vi "synnax writer open.vi"(4 "enable_auto_commit (F)":bool, 5 "err_on_unauthorized (F)":bool, 6 "auto_index (F)":bool, 7 "start (now)":timestamp, 8 "error in":errorcluster, 9 "authorities (255 for all channels)":u8[](array[numeric]), 10 "channels":u32[](array[numeric]), 11 "sy client handle":u64) -> (0 "error out":errorcluster, 2 "channels out":u32[](array[numeric]), 3 "sy writer handle":u64)   [LabVIEW 2026, in "synnax_clib.lvlib" / "Synnax Writer.lvclass"]
doc: "SYNNAX_EXPORT int32_t synnax_writer_open(\n SynnaxClient client,\n int64_t start,\n const uint32_t *channels,\n uint64_t channel_count,\n int32_t mode,\n int32_t enable_auto_commit,\n SynnaxWriter *out_writer,\n SynnaxError err\n);"
uses:
  Synnax Writer.lvclass
  typedefs/writer_mode.ctl
  subvis/Timestamp Conversion Single.vi
  Synnax Writer.lvclass/Synnax Writer.ctl
  synnax_clib.lvlib
  synnax_clib.dll
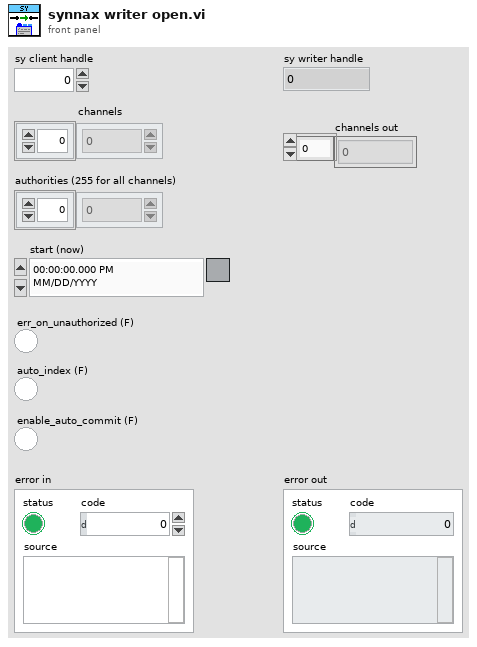
[diagram p1: front panel]
types:
  T1 = typedef "synnax_clib.lvlib/writer_mode.ctl" = enum16{"PERSIST & STREAM", "PERSIST", "STREAM"}
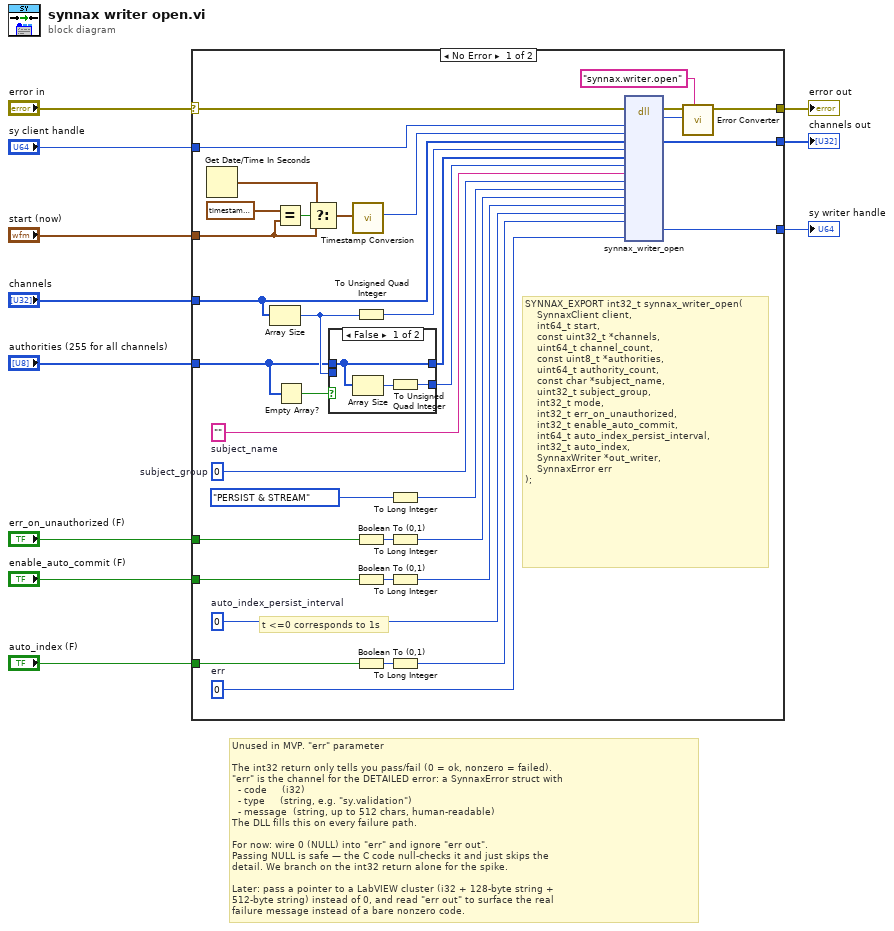
[diagram p0: block diagram]
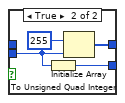
[diagram p2: hidden frame]
diagram:
  # "Unused in MVP. \"err\" parameter\n\nThe int32 return only tells you pass/fail (0 = ok, nonzero = failed).\n\"err\" is the channel for the DETAILED error: a SynnaxError struct with\n  - code     (i32)\n  - type     (string, e.g. \"sy.validation\")\n  - message  (string, up to 512 chars, human-readable)\nThe DLL fills this on every failure path.\n\nFor now: wire 0 (NULL) into \"err\" and ignore \"err out\".\nPassing NULL is safe — the C code null-checks it and just skips the\ndetail. We branch on the int32 return alone for the spike.\n\nLater: pass a pointer to a LabVIEW cluster (i32 + 128-byte string +\n512-byte string) instead of 0, and read \"err out\" to surface the real\nfailure message instead of a bare nonzero code."
  n1 = case shown="No Error" "error in" {
    selector: "error in" -> [w15 w55]
    tunnel: "enable_auto_commit (F)" -> [w47 _]
    tunnel: [w43 w55] -> w10
    tunnel: "err_on_unauthorized (F)" -> [w38 _]
    tunnel: "auto_index (F)" -> [w34 _]
    tunnel: "authorities (255 for all channels)" -> [w27 _]
    tunnel: "start (now)" -> [w13 _]
    tunnel: [w22 _] -> w5
    tunnel: [w21 _] -> w4
    tunnel: "channels" -> [w20 _]
    tunnel: "sy client handle" -> [w19 _]
    frame No Error {
      w35 = i64 0  # auto_index_persist_interval
      w39 = u32 0  # subject_group
      w40 = ""  # subject_name
      w45 = u64 0  # err
      # "t <=0 corresponds to 1s"
      # "SYNNAX_EXPORT int32_t synnax_writer_open(\n    SynnaxClient client,\n    int64_t start,\n    const uint32_t *channels,\n    uint64_t channel_count,\n    const uint8_t *authorities,\n    uint64_t authority_count,\n    const char *subject_name,\n    uint32_t subject_group,\n    int32_t mode,\n    int32_t err_on_unauthorized,\n    int32_t enable_auto_commit,\n    int64_t auto_index_persist_interval,\n    int32_t auto_index,\n    SynnaxWriter *out_writer,\n    SynnaxError err\n);"
      n2 = Get Date/Time In Seconds() -> (seconds since 1Jan1904=w14:timestamp)
      n3 = Array Size(array=w20) -> (size(s)=w30:i32)
      n4 = Equal?(x=timestamp timestamp(0 s since 1904-01-01), y=w13) -> (x = y?=w25:bool)
      n5 = Empty Array?(array=w27) -> (empty?=w28:bool)
      n6 = Select(t=w14, s=w25, f=w13) -> (s? t:f=w24:timestamp)
      n7 = case shown="False" w28 {
        tunnel: [w49 w54] -> w31
        tunnel: w30 -> [_ w52]
        tunnel: w27 -> [w49 _]
        tunnel: [w48 w51] -> w26
        frame False {
          n8 = Array Size(array=w49) -> (size(s)=w50:i32)
          n9 = To Unsigned Quad Integer(1:w50) -> (0:w48:u64)
        }
        frame True {
          n10 = To Unsigned Quad Integer(1:w52) -> (0:w51:u64)
          n11 = Initialize Array(u8 255, w52) -> (w54:u8[])
        }
      }
      n12 = call-poly "Timestamp Conversion.vi"("timestamp"=w24) -> ("timestamp (ns)"=w23:i64)  [unwired: 9 in]
      n13 = To Unsigned Quad Integer(1:w30) -> (0:w29:u64)
      n14 = Boolean To (0,1)(Boolean=w38) -> (0, 1=w37:i16)
      n15 = Boolean To (0,1)(Boolean=w47) -> (0, 1=w46:i16)
      n16 = Boolean To (0,1)(Boolean=w34) -> (0, 1=w33:i16)
      n17 = To Long Integer(number=writer_mode."PERSIST & STREAM") -> (32bit integer=w41:i32)
      n18 = To Long Integer(number=w37) -> (32bit integer=w36:i32)
      n19 = To Long Integer(number=w46) -> (32bit integer=w44:i32)
      n20 = To Long Integer(number=w33) -> (32bit integer=w32:i32)
      n21 = dll-call lib="C/synnax/client/labview/synnax_clib.*" fn="synnax_writer_open"(error in=w15, "client"=w19, "start"=w23, "channels"=w20, "channel_count"=w29, "authorities"=w31, "authority_count"=w26, "subject_name"=w40, "subject_group"=w39, "mode"=w41, "err_on_unauthorized"=w36, "enable_auto_commit"=w44, "auto_index_persist_interval"=w35, "auto_index"=w32, "err"=w45) -> (error out=w18:errorcluster, "return type"=w17:i32, "channels"=w22:u32[], "out_writer"=w21:u64)  [unwired: 16 in, 1 out]
      n22 = call "Error Converter.vi"("source"="synnax.writer.open", "error code"=w17, "error in (no error)"=w18) -> ("error out"=w43:errorcluster)  [unwired: 8 in]
    }
    frame Error {
    }
  }
  "error out" <- w10
  "channels out" <- w5
  "sy writer handle" <- w4
